vi "Up_ExposureAndGain.vi"(8 "error in (no error)":errorcluster, 9 "Expouse":refnum<vi>, 10 "Gain":refnum<vi>, 11 "Session Out":T1) -> (0 "error out":errorcluster)   [LabVIEW 2019]
uses:
  <vilib>/userdefined/High Color/IMAQdx.ctl
  <resource>/objmgr/imaqdx.rc
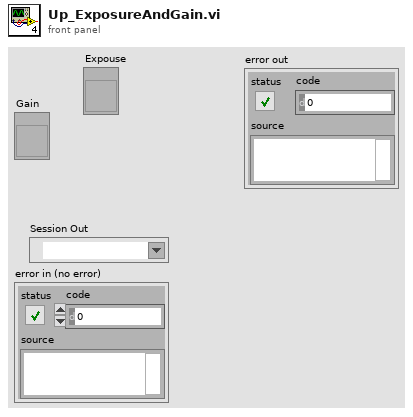
[diagram p1: front panel]
types:
  T1 = typedef "IMAQdx.ctl" = refnum<k21>
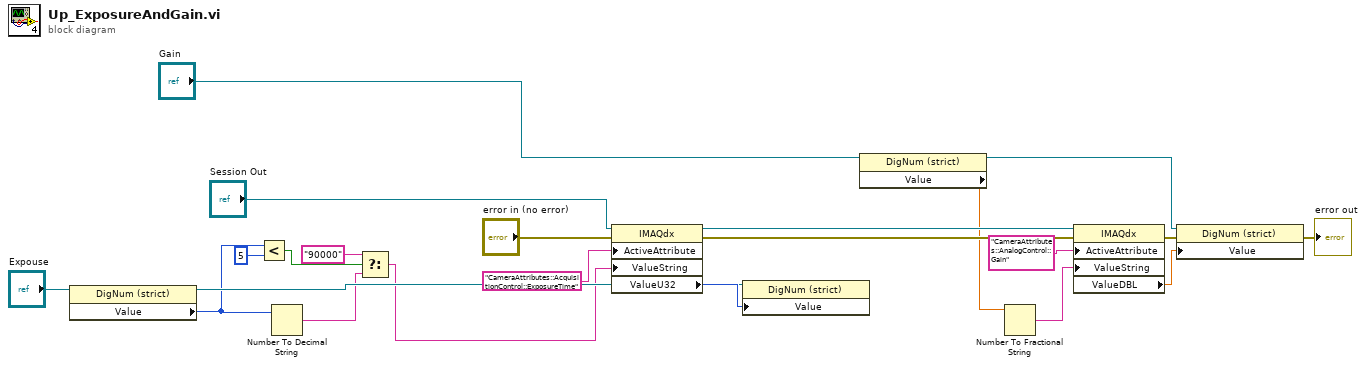
[diagram p0: block diagram]
diagram:
  n1 = property class="DigNum (strict)"(reference="Expouse") -> (reference out=w15:refnum<vi>, "Value"=w6:u32)  [unwired: 1 in, 1 out]
  n2 = Less?(x=w6, y=u32 5) -> (x < y?=w4:bool)
  n3 = Number To Decimal String(number=w6) -> (decimal integer string=w3:string)  [unwired: 1 in]
  n4 = Select(t="90000", s=w4, f=w3) -> (s? t:f=w1:string)
  n5 = property class="IMAQdx"(reference="Session Out", error in="error in (no error)", "ActiveAttribute"="CameraAttributes::AcquisitionControl::ExposureTime", "ValueString"=w1) -> (reference out=w19:T1, error out=w11:errorcluster, "ValueU32"=w22:u32)
  n6 = property class="DigNum (strict)"(reference=w15, "Value"=w22) -> ()  [unwired: 1 in, 2 out]
  n7 = property class="DigNum (strict)"(reference="Gain") -> (reference out=w13:refnum<vi>, "Value"=w7:dbl)  [unwired: 1 in, 1 out]
  n8 = Number To Fractional String(number=w7) -> (F-format string=w17:string)  [unwired: 3 in]
  n9 = property class="IMAQdx"(reference=w19, error in=w11, "ActiveAttribute"="CameraAttributes::AnalogControl::Gain", "ValueString"=w17) -> (error out=w10:errorcluster, "ValueDBL"=w12:dbl)  [unwired: 1 out]
  n10 = property class="DigNum (strict)"(reference=w13, error in=w10, "Value"=w12) -> (error out=→"error out":errorcluster)  [unwired: 1 out]
